vi "Get ID.vi"(8 "error in (no error)":errorcluster, 10 "id":i32, 11 "devNum":i32) -> (0 "error out":errorcluster, 2 "id out":i32, 3 "function return":u32)   [LabVIEW 2014, in "atmcd32d.lvlib"]
doc: "unsigned int WINAPI GetID(int devNum, int * id);"
uses:
  atmcd32d.lvlib
  atmcd32d.dll
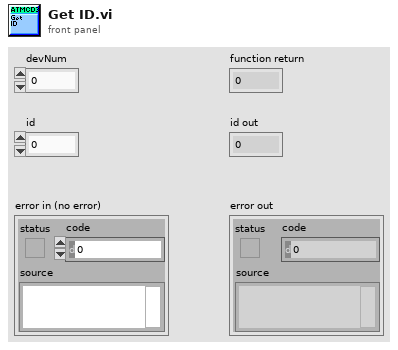
[diagram p1: front panel]
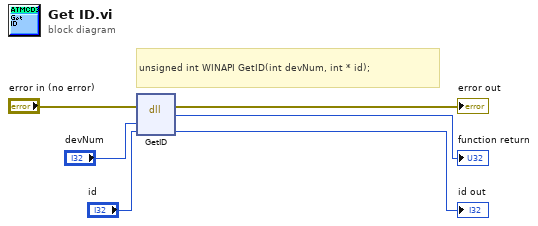
[diagram p0: block diagram]
diagram:
  # "unsigned int WINAPI GetID(int devNum, int * id);"
  n1 = dll-call lib="C:/Users/Bakir/Documents/Lambda2-Testing/lib/Andorlib/atmcd32d.*" fn="GetID"(error in="error in (no error)", "devNum"="devNum", "id"="id") -> (error out=→"error out":errorcluster, →"function return":u32, "id"=→"id out":i32)  [unwired: 3 in, 1 out]
